vi "CSTK_Icon_Creator_Insert_OpenTemplate.vi"(8 "错误输入（无错误）":errorcluster, 11 "模板相对路径":string) -> (0 "错误输出":errorcluster, 3 "图片输出":picture, 4 "图片数据输出":T1)   [LabVIEW 2015, in "CSTK_Icon Creator.lvlib"]
uses:
  CSTK_Icon Creator.lvlib
  <vilib>/picture/picture.llb/imagedata.ctl
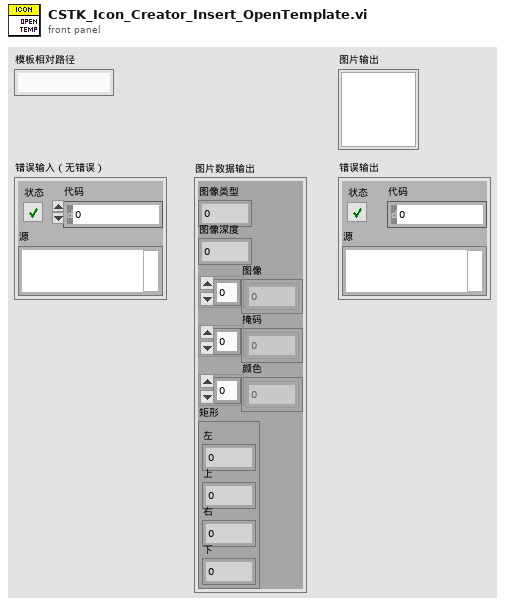
[diagram p1: front panel]
types:
  T1 = typedef "imagedata.ctl" = cluster{"image type":i32, "image depth":i32, "image":u8[], "mask":u8[], "colors":u32[], "Rectangle":cluster{"left":i16, "top":i16, "right":i16, "bottom":i16}}
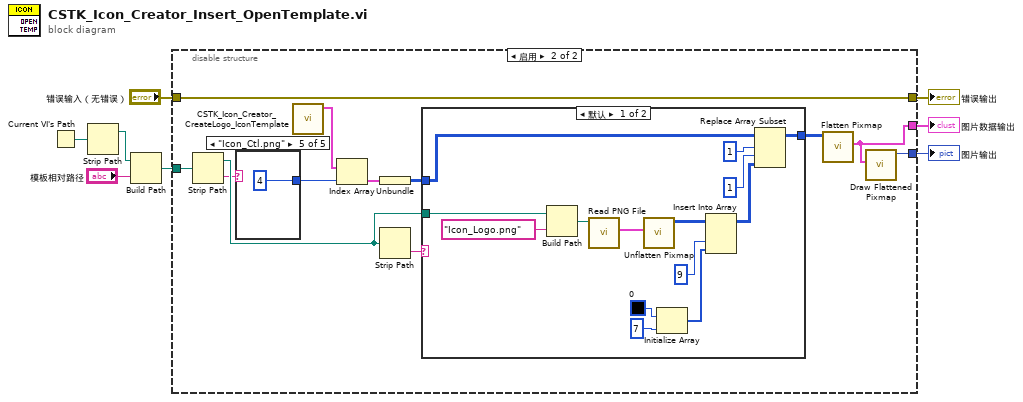
[diagram p0: block diagram]
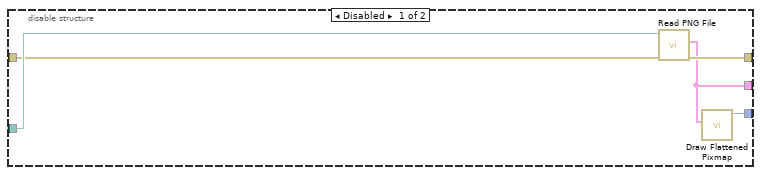
[diagram p2: hidden frame]
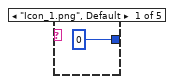
[diagram p4: hidden frame]
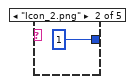
[diagram p5: hidden frame]
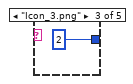
[diagram p6: hidden frame]
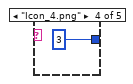
[diagram p7: hidden frame]
diagram:
  n1 = Current VI's Path() -> (path=w5:path)
  n2 = Strip Path(path=w5) -> (stripped path=w6:path)  [unwired: 1 out]
  n3 = Build Path(base path=w6, name or relative path="模板相对路径") -> (appended path=w8:path)
  n4 = disable-structure shown="启用" {
    disable-tunnel: w8 -> [w13 w25]
    disable-tunnel: [w12 w20] -> w4
    disable-tunnel: "错误输入（无错误）" -> [w11 w20]
    disable-tunnel: [w10 w21] -> w2
    disable-tunnel: [w9 w22] -> w1
    frame Disabled {
      n5 = call <vilib>:"Read PNG File.vi"("error in (no error)"=w11, "path to PNG file"=w13) -> ("error out"=w12:errorcluster, "image data"=w10:T1)  [unwired: 7 in, 1 out]
      n6 = call <vilib>:"Draw Flattened Pixmap.vi"("image data"=w10) -> ("new picture"=w9:picture)  [unwired: 8 in]
    }
    frame Enabled {
      n7 = Strip Path(path=w25) -> (stripped path=w24:path, name=w23:string)
      n8 = case shown="\"Icon_Ctl.png\"" w23 {
        tunnel: [0 1 2 3 4] -> w18
        frame "Icon_1.png", Default {
        }
        frame "Icon_2.png" {
        }
        frame "Icon_3.png" {
        }
        frame "Icon_4.png" {
        }
        frame "Icon_Ctl.png" {
        }
      }
      n9 = call "CSTK_Icon_Creator_CreateLogo_IconTemplate.vi"() -> ("Icon Template"=w19:cluster{"Icon_Ctl":u32[][]}[])  [unwired: 11 in]
      n10 = Index Array(array=w19, index=w18) -> (element=w16:cluster{"Icon_Ctl":u32[][]})
      n11 = Unbundle(w16) -> ("Icon_Ctl"=w17:u32[][])
      n12 = Strip Path(path=w24) -> (name=w14:string)  [unwired: 1 out]
      n13 = case shown="默认" w14 {
        tunnel: w24 -> [w39 _]
        tunnel: w17 -> [w30 w40]
        tunnel: [w26 w40] -> w15
        frame Default {
          n14 = Build Path(base path=w39, name or relative path="Icon_Logo.png" ("名称或相对路径")) -> (appended path=w37:path)
          n15 = call <vilib>:"Read PNG File.vi"("path to PNG file"=w37) -> ("image data"=w36:T1)  [unwired: 8 in, 2 out]
          n16 = call <vilib>:"Unflatten Pixmap.vi"("image data"=w36) -> ("24-bit pixmap"=w27:u32[][])  [unwired: 4 in, 6 out]
          n17 = Initialize Array(u32 0, 7 ("维数大小")) -> (w31:u32[])
          n18 = Insert Into Array(array=w27, index (col)=9 ("禁用的索引 (列)"), new element=w31) -> (w35:u32[][])  [unwired: 1 in]
          n19 = Replace Array Subset(array=w30, new element=w35, index (row)=1 ("索引 (行)"), index (col)=1 ("禁用的索引 (列)")) -> (w26:u32[][])
        }
        frame "Default" {
        }
      }
      n20 = call <vilib>:"Flatten Pixmap.vi"("24-bit pixmap"=w15) -> ("image data"=w21:T1)  [unwired: 10 in]
      n21 = call <vilib>:"Draw Flattened Pixmap.vi"("image data"=w21) -> ("new picture"=w22:picture)  [unwired: 8 in]
    }
  }
  "错误输出" <- w4
  "图片数据输出" <- w2
  "图片输出" <- w1
